vi "NF WF1973_74 CHAN Delt.vi"(0 "VISAsession":refnum<visa-resource-name>, 5 "Set Frequency(Input)":u16(ring) caption="Set FrequencyInput)" items=["Input", "Minimum", "Maximum"], 7 "Frequency(0)":dbl format="%.8f", 9 "Units(Hz)":i32(slide)=2 min=0 max=4 step=1 scale=0.0..4.0, 11 "error in (no error)":errorcluster caption="Error IN", 12 "Read(F)":bool) -> (4 "CopyVISAsession":refnum<visa-resource-name>, 6 "Query Frequency":dbl format="%.8f", 15 "error out":errorcluster caption="Error OUT")   [LabVIEW 2010]
panel:
  # "n[Hz]"
  # "Choose\nInput"
  # "u[Hz]"
  # "[Hz]"
  # "k[Hz]"
  # "M[Hz]"
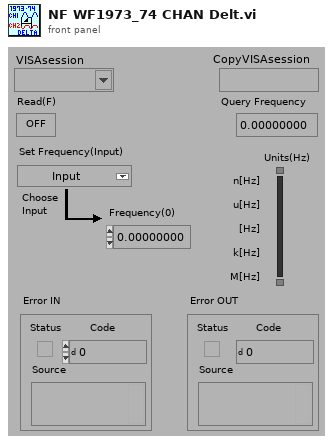
[diagram p1: front panel]
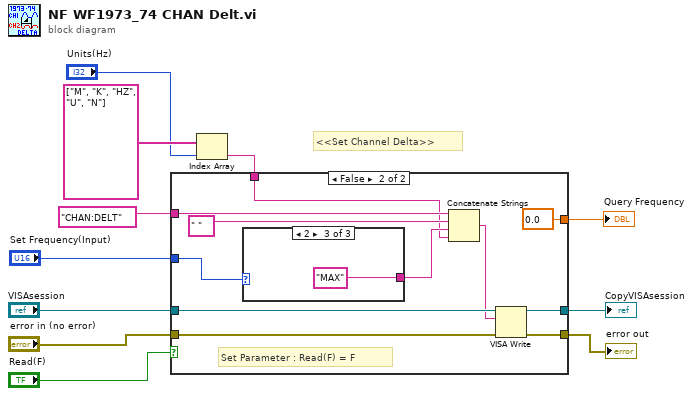
[diagram p0: block diagram]
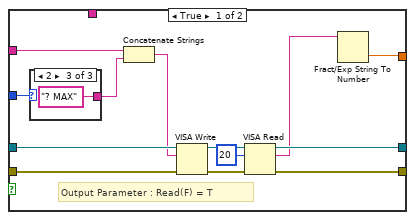
[diagram p2: hidden frame]
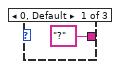
[diagram p3: hidden frame]
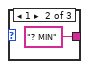
[diagram p4: hidden frame]
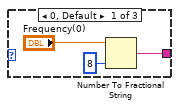
[diagram p5: hidden frame]
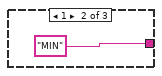
[diagram p6: hidden frame]
diagram:
  # "<<Set Channel Delta>>"
  n1 = Index Array(array=string[] ["M", "K", "HZ", "U", "N"], index="Units(Hz)") -> (element=w3:string)
  n2 = case shown="FALSE" "Read(F)" {
    tunnel: "VISAsession" -> [w24 w38]
    tunnel: [w21 w35] -> w10
    tunnel: [w20 w36] -> w9
    tunnel: "error in (no error)" -> [w19 w37]
    tunnel: "CHAN:DELT" ("文字列") -> [w17 w32]
    tunnel: [w15 0.0] -> w5
    tunnel: w3 -> [_ w30]
    tunnel: "Set Frequency(Input)" -> [w13 w28]
    frame True {
      # "Output Parameter : Read(F) = T"
      n3 = case shown="2" w13 {
        tunnel: ["?" ("形式文字列") "? MIN" ("形式文字列") "? MAX" ("形式文字列")] -> w12
        frame 0, Default {
        }
        frame 1 {
        }
        frame 2 {
        }
      }
      n4 = Concatenate Strings(w17, w12) -> (w16:string)
      n5 = VISA Write(VISA resource name=w24, write buffer=w16, error in (no error)=w19) -> (VISA resource name out=w22:refnum<visa-resource-name>, error out=w23:errorcluster)  [unwired: 1 out]
      n6 = VISA Read(VISA resource name=w22, byte count=u32 20 ("バイトカウント（0）"), error in (no error)=w23) -> (VISA resource name out=w21:refnum<visa-resource-name>, read buffer=w14:string, error out=w20:errorcluster)  [unwired: 1 out]
      n7 = Fract/Exp String To Number(string=w14) -> (number=w15:dbl)  [unwired: 3 in, 1 out]
    }
    frame False {
      # "Set Parameter : Read(F) = F"
      n8 = case shown="2" w28 {
        tunnel: [w39 "MIN" "MAX"] -> w31
        frame 0, Default {
          n9 = Number To Fractional String(number="Frequency(0)", precision (6)=i16 8 ("精度 (6)")) -> (F-format string=w39:string)  [unwired: 2 in]
        }
        frame 1 {
        }
        frame 2 {
        }
      }
      n10 = Concatenate Strings(w32, " ", w31, w30) -> (w34:string)
      n11 = VISA Write(VISA resource name=w38, write buffer=w34, error in (no error)=w37) -> (VISA resource name out=w35:refnum<visa-resource-name>, error out=w36:errorcluster)  [unwired: 1 out]
    }
  }
  "error out" <- w9
  "CopyVISAsession" <- w10
  "Query Frequency" <- w5
